vi "Initialize.vi"(7 "Baud Rate":u32(ring)=5 items=["<0>"=0, "4800"=4800, "9600"=9600, "19200"=19200, "38400"=38400, "57600"=57600, "115200"=115200], 8 "error in (no error)":errorcluster, 9 "ID Query (True)":bool=TRUE, 10 "Reset (True)":bool=TRUE, 11 "VISA resource name":refnum<visa-resource-name>) -> (0 "error out":errorcluster, 3 "VISA resource name out":refnum<visa-resource-name>, 5 "*IDN?":string)   [LabVIEW 2020]
doc: "Establishes communication with the instrument and optionally performs an instrument identification query and/or an instrument reset. It also places the instrument in a default state needed for other instrument driver operations. Therefore, call this VI before calling other instrument driver VIs for this instrument. Generally, you need to call the Initialize VI only once at the beginning of an application."
uses:
  <instrlib>/BK Precision 911X Series/BK Precision 911X Series.lvlib
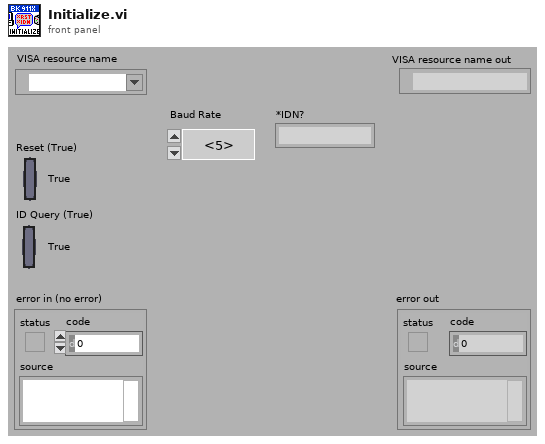
[diagram p1: front panel]
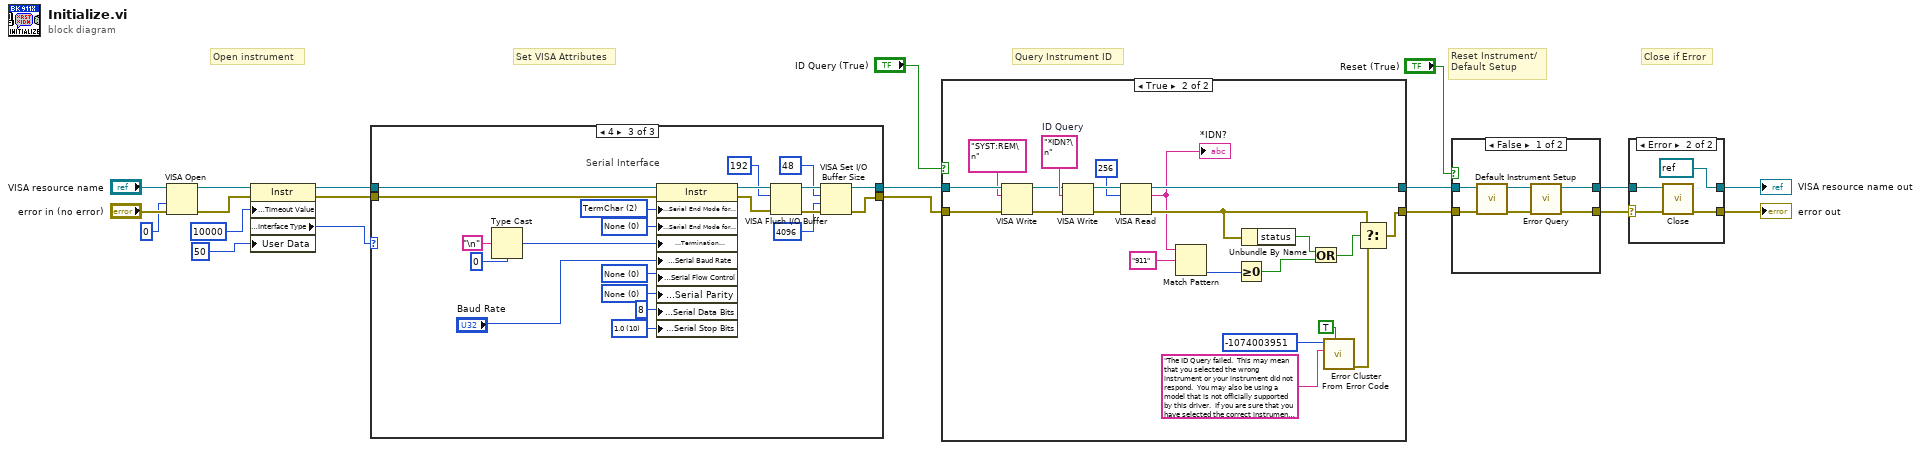
[diagram p0: block diagram]
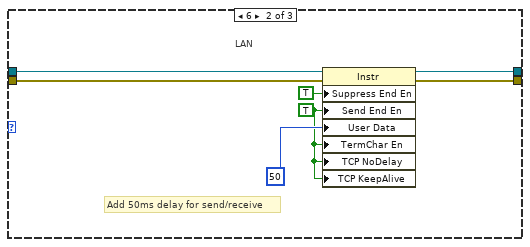
[diagram p3: hidden frame]
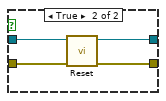
[diagram p5: hidden frame]
diagram:
  # "Set VISA Attributes"
  # "Close if Error"
  # "Query Instrument ID"
  # "Reset Instrument/\nDefault Setup"
  # "Open instrument"
  n1 = VISA Open(access mode=u32 0, error in (no error)="error in (no error)", VISA resource name="VISA resource name") -> (VISA resource name=w4:refnum<visa-resource-name>, error out=w3:errorcluster)  [unwired: 2 in]
  n2 = property class="Instr"(reference=w4, error in=w3, "General Settings:Timeout Value"=u32 10000, "User Data"=u32 50 ("General Settings:User Data")) -> (reference out=w11:refnum<visa-resource-name>, error out=w10:errorcluster, "Interface Information:Interface Type"=w2:u16)
  n3 = case shown="4" w2 {
    tunnel: [w22 w25 w47] -> w13
    tunnel: [w21 w26 w44] -> w12
    tunnel: w11 -> [w22 w28 w49]
    tunnel: w10 -> [w21 w27 w50]
    frame 1, 7, Default {
      # "USBTMC and GPIB"
    }
    frame 6 {
      w23 = TRUE ("Message Based Settings:Send End Enable")
      # "Add 50ms delay for send/receive"
      # "LAN"
      n4 = property class="Instr"(reference=w28, error in=w27, "Suppress End En"=TRUE ("Message Based Settings:Suppress End Enable"), "Send End En"=w23, "User Data"=u32 50, "TermChar En"=w23, "TCP NoDelay"=w23, "TCP KeepAlive"=w23) -> (reference out=w25:refnum<visa-resource-name>, error out=w26:errorcluster)
    }
    frame 4 {
      w31 = u16 0 items=["None", "XON/XOFF", "RTS/CTS", "XON/XOFF & RTS/CTS", "DTR/DSR", "XON/XOFF & DTR/DSR"] ("Serial Settings:Flow Control")
      w32 = u16 0 items=["None", "Odd", "Even", "Mark", "Space"] ("Serial Settings:Parity")
      w34 = u16 10 items=["1.0"=10, "1.5"=15, "2.0"=20] ("Serial Settings:Stop Bits")
      w35 = u16 0 items=["None", "Last Bit", "TermChar", "Break"] ("Serial Settings:End Mode for Writes")
      w37 = u16 2 items=["None", "LastBit", "TermChar"] ("Termination Character")
      # "Serial Interface"
      n5 = Type Cast(type=u8 0, x="\n" ("Line Feed Constant")) -> (*(type *) &x=w36:u8)
      n6 = property class="Instr"(reference=w49, error in=w50, "Serial Settings:Serial End Mode for Reads"=w37, "Serial Settings:Serial End Mode for Writes"=w35, "Message Based Settings:Termination Character"=w36, "Serial Settings:Serial Baud Rate"="Baud Rate", "Serial Settings:Serial Flow Control"=w31, "Serial Settings:Serial Parity"=w32, "Serial Settings:Serial Data Bits"=u16 8 ("Serial Settings:Data Bits"), "Serial Settings:Serial Stop Bits"=w34) -> (reference out=w43:refnum<visa-resource-name>, error out=w46:errorcluster)
      n7 = VISA Flush I/O Buffer(VISA resource name=w43, mask (16)=u16 192, error in (no error)=w46) -> (VISA resource name out=w48:refnum<visa-resource-name>, error out=w45:errorcluster)
      n8 = VISA Set I/O Buffer Size(VISA resource name=w48, mask (16)=u16 48, size (4096)=u32 4096 ("size (0)"), error in (no error)=w45) -> (VISA resource name out=w47:refnum<visa-resource-name>, error out=w44:errorcluster)
    }
  }
  n9 = case shown="True" "ID Query (True)" {
    tunnel: [w51 w74] -> w19
    tunnel: [w52 w73] -> w20
    tunnel: w13 -> [w52 w56]
    tunnel: w12 -> [w51 w55]
    frame False {
    }
    frame True {
      w68 = "*IDN?\n"  # ID Query
      n10 = VISA Write(VISA resource name=w56, write buffer="SYST:REM\n", error in (no error)=w55) -> (VISA resource name out=w57:refnum<visa-resource-name>, error out=w58:errorcluster)  [unwired: 1 out]
      n11 = VISA Write(VISA resource name=w57, write buffer=w68, error in (no error)=w58) -> (VISA resource name out=w72:refnum<visa-resource-name>, error out=w71:errorcluster)  [unwired: 1 out]
      n12 = VISA Read(VISA resource name=w72, byte count=u32 256, error in (no error)=w71) -> (VISA resource name out=w73:refnum<visa-resource-name>, read buffer=w53:string, error out=w62:errorcluster)  [unwired: 1 out]
      "*IDN?" <- w53
      n13 = Match Pattern(string=w53, regular expression="911") -> (offset past match=w63:i32)  [unwired: 1 in, 3 out]
      n14 = Greater Or Equal To 0?(x=w63) -> (x >= 0?=w60:bool)
      n15 = Unbundle By Name(w62) -> ("status"=w61:bool)
      n16 = Or(x=w61, y=w60) -> (x .or. y?=w59:bool)
      n17 = call <vilib>:"Error Cluster From Error Code.vi"("show call chain? (False)"=TRUE, "error message (\"\")"="The ID Query failed.  This may mean that you selected the wrong instrument or your instrument did not respond.  You may also be using a model that is not officially supported by this driver.  If you are sure that you have selected the correct instrument and it is responding, try disabling the ID Query." ("Source (VI Name)"), "error code (0)"=-1074003951 ("Code")) -> ("error out"=w67:errorcluster)  [unwired: 6 in]
      n18 = Select(t=w62, s=w59, f=w67) -> (s? t:f=w74:errorcluster)
    }
  }
  n19 = case shown="False" "Reset (True)" {
    tunnel: w19 -> [w78 w81]
    tunnel: [w79 w84] -> w5
    tunnel: w20 -> [w77 w82]
    tunnel: [w80 w83] -> w6
    frame False {
      n20 = call "Default Instrument Setup.vi"("error in (no error)"=w78, "VISA resource name"=w77) -> ("error out"=w76:errorcluster, "VISA resource name out"=w75:refnum<visa-resource-name>)  [unwired: 8 in]
      n21 = call <instrlib>:"Error Query.vi"("error in (no error)"=w76, "VISA resource name"=w75) -> ("error out"=w79:errorcluster, "VISA resource name out"=w80:refnum<visa-resource-name>)  [unwired: 6 in, 2 out]
    }
    frame True {
      n22 = call <instrlib>:"Reset.vi"("error in (no error)"=w81, "VISA resource name"=w82) -> ("error out"=w84:errorcluster, "VISA resource name out"=w83:refnum<visa-resource-name>)  [unwired: 8 in]
    }
  }
  n23 = case shown="Error" w5 {
    selector: w5 -> [w85 w88]
    tunnel: w6 -> [w86 w89]
    tunnel: [w86 refnum<visa-resource-name> refnum ("VISA resource name out")] -> w8
    tunnel: [w85 w90] -> w7
    frame No Error {
    }
    frame Error {
      n24 = call <instrlib>:"Close.vi"("error in (no error)"=w88, "VISA resource name"=w89) -> ("error out"=w90:errorcluster)  [unwired: 9 in]
    }
  }
  "VISA resource name out" <- w8
  "error out" <- w7
